vi "Restore Configuration.vi"(8 "error in (no error)":errorcluster, 9 "Initialization":bool, 10 "File path":path, 11 "Measure Object in":refnum<class "NHMFL Synthesizer.lvclass">) -> (0 "error out":errorcluster, 1 "Section out":string, 2 "File path out":path, 3 "Measure Object out":refnum<class "NHMFL Synthesizer.lvclass">)   [LabVIEW 2021, in "NHMFL Synthesizer.lvclass"]
uses:
  NHMFL Synthesizer.lvclass
  NHMFL Synthesizer.lvclass/NHMFL Synthesizer.ctl
  Process Object/Process Object.lvclass
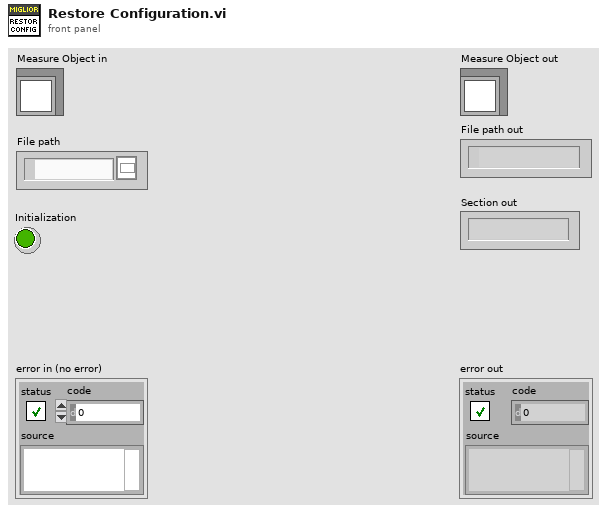
[diagram p1: front panel]
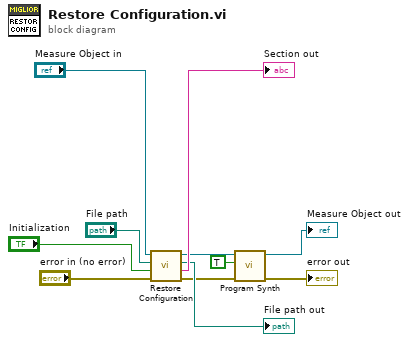
[diagram p0: block diagram]
diagram:
  n1 = call-parent "Restore Configuration.vi"("error in (no error)"="error in (no error)", "Initialization"="Initialization", "File path"="File path", "Measure Object in"="Measure Object in") -> ("error out"=w6:errorcluster, "Section out"=→"Section out":string, "File path out"=→"File path out":path, "Measure Object out"=w5:refnum<class "NHMFL Synthesizer.lvclass">)  [unwired: 4 in]
  n2 = call-dynamic "Program Synth.vi"("error in (no error)"=w6, "Check if valid device"=TRUE, "NHMFL Synthesizer in"=w5) -> ("error out"=→"error out":errorcluster, "NHMFL Synthesizer out"=→"Measure Object out":refnum<class "NHMFL Synthesizer.lvclass">)  [unwired: 7 in]
